vi "Channel_Status.vi"(8 "error in":errorcluster, 10 "Channel":string, 11 "MLTFNC in":refnum<class "MLTFNC.lvclass">) -> (0 "error out":errorcluster, 2 "Routed":bool, 3 "MLTFNC out":refnum<class "MLTFNC.lvclass">)   [LabVIEW 2019, in "MLTFNC.lvlib" / "MLTFNC.lvclass"]
uses:
  Library/MLTFNC.lvclass
  Library/MLTFNC.lvclass/MLTFNC.ctl
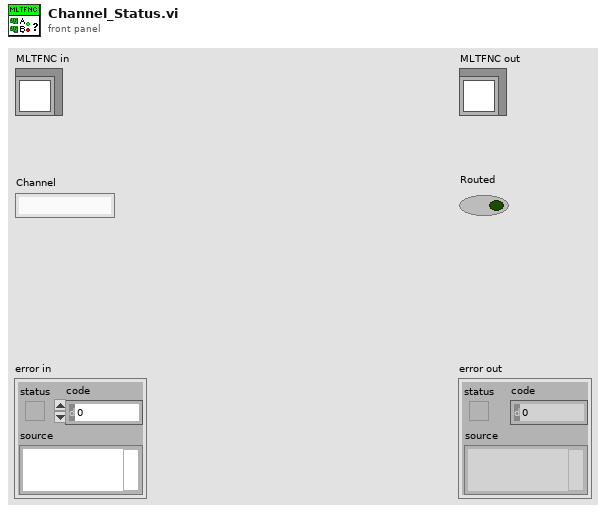
[diagram p1: front panel]
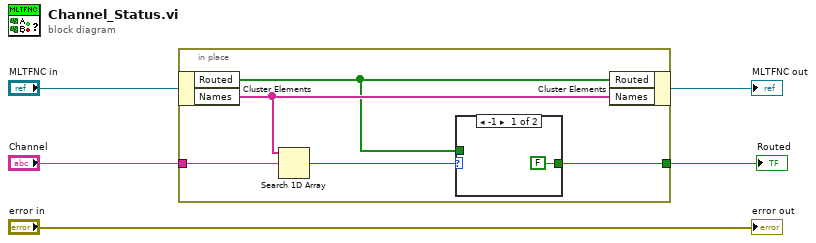
[diagram p0: block diagram]
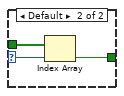
[diagram p2: hidden frame]
diagram:
  n1 = in-place {
    in-place-border: "Channel" -> [w9]
    in-place-border: [w7] -> w2
    n2 = in-place-cluster #1("MLTFNC in") -> ("Routed"=w8:bool[], "Names"=w10:string[])
    n3 = Search 1D Array(1D array=w10, element=w9) -> (index of element=w6:i32)  [unwired: 1 in]
    n4 = case shown="-1" w6 {
      selector: w6 -> [_ w12]
      tunnel: w8 -> [_ w14]
      tunnel: [FALSE ("Boolean") w13] -> w7
      frame -1 {
      }
      frame Default {
        n5 = Index Array(array=w14, index=w12) -> (element=w13:bool)
      }
    }
    n6 = in-place-cluster #1("Routed"=w8, "Names"=w10) -> (→"MLTFNC out":refnum<class "MLTFNC.lvclass">)
  }
  "Routed" <- w2
  "error out" <- "error in"
